vi "SQL查询.vi"(7 "condition":string, 10 "table输入":string(combo), 11 "database":string(combo)) -> (0 "error out":errorcluster, 3 "data":string[][](table))   [LabVIEW 2016, in "数据传输系统.lvlib"]
uses:
  <vilib>/Utility/sysdir.llb/System Directory Type.ctl
  <vilib>/addons/database/Connection.llb/DB Tools Open Connec (String).vi
  <vilib>/addons/database/_DB Variant To Data/Database Variant To Data.xnode
  <vilib>/addons/database/NI_Database_API.lvlib
panel:
  out "子数组":string[](array[string])
  in  "error in (no error)":errorcluster
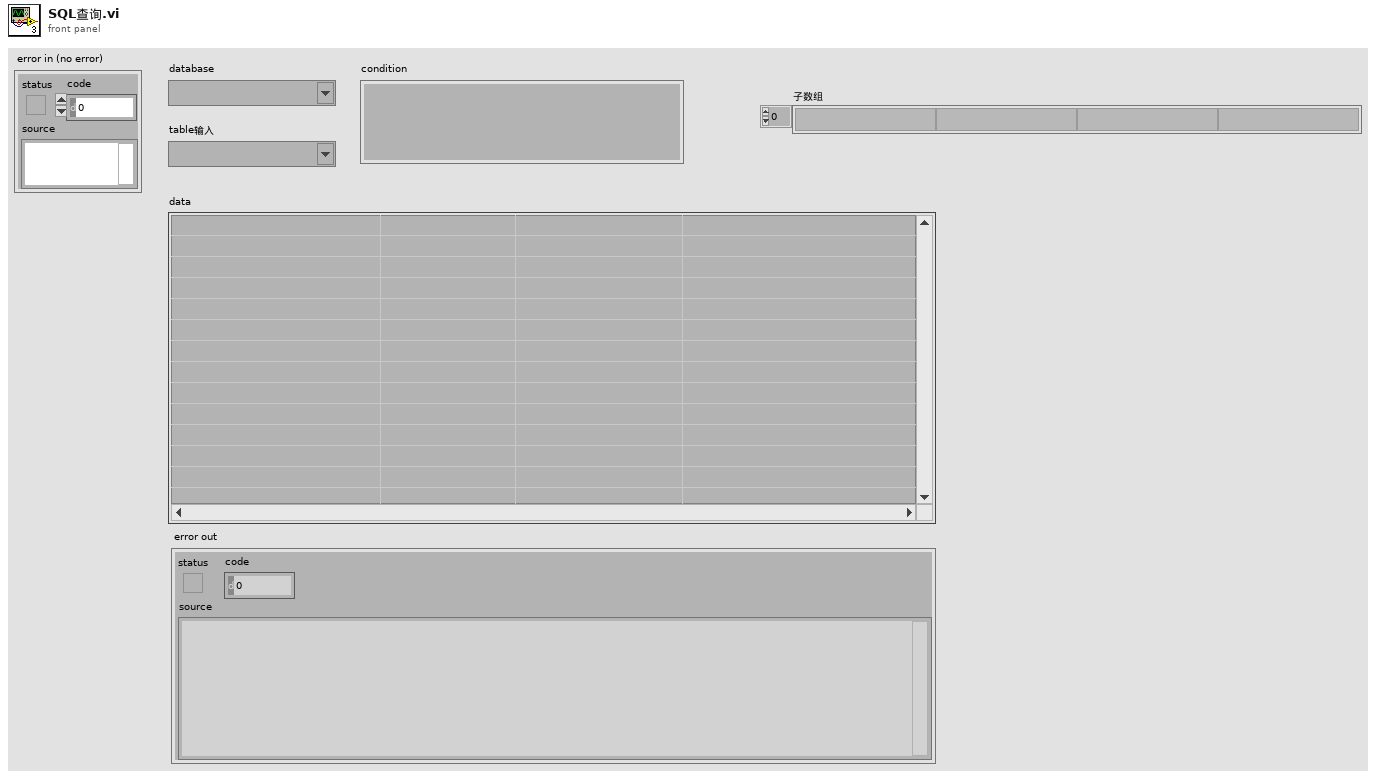
[diagram p1: front panel]
types:
  T1 = typedef "System Directory Type.ctl" = i32
  T2 = typedef "NI_Database_API.lvlib/Conn ObjectReference.ctl" = refnum<k1>
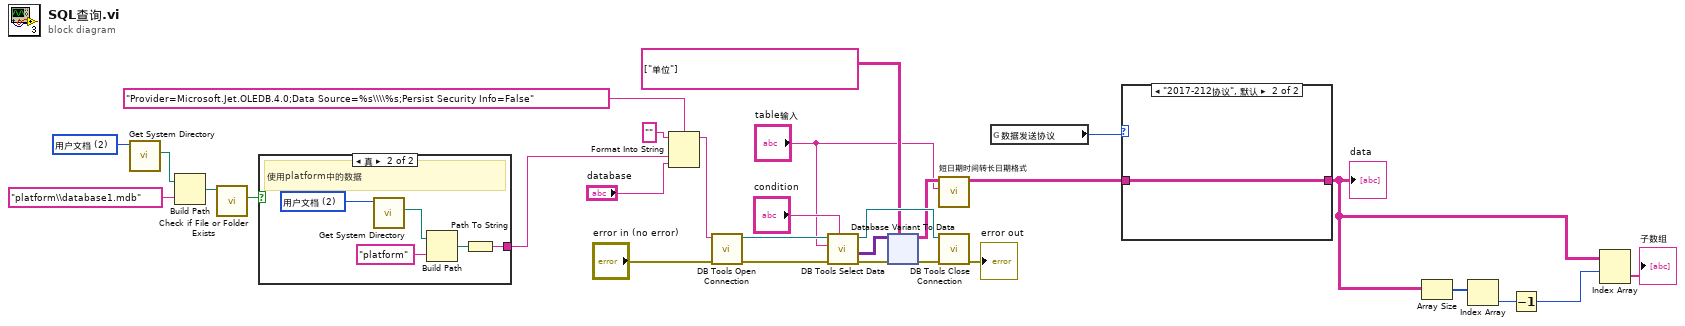
[diagram p0: block diagram]
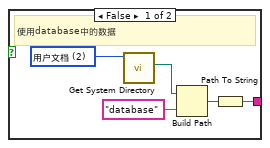
[diagram p2: hidden frame]
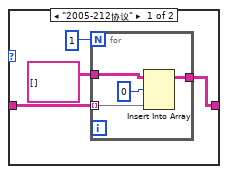
[diagram p3: hidden frame]
diagram:
  w5 = T1 2 items=["用户目录"=0, "用户桌面"=1, "用户文档"=2, "用户应用程序数据"=3, "用户设置"=4, "用户临时目录"=5, "公共文档"=6, "公共应用程序数据"=7, "公共设置"=8, "公共缓存"=13, "系统核心库"=9, "系统安装库"=10, "应用程序文件"=11, "启动盘根目录"=12] ("system directory type")
  n1 = call <vilib>:"Get System Directory.vi"("system directory type"=w5) -> ("system directory"=w6:path)  [unwired: 10 in]
  n2 = Build Path(base path=w6, name or relative path="platform\\database1.mdb" ("condition")) -> (appended path=w4:path)
  n3 = call <vilib>:"Check if File or Folder Exists.vi"("path"=w4) -> ("file or folder exists?"=w2:bool)  [unwired: 8 in, 2 out]
  n4 = case shown="真" w2 {
    tunnel: [w30 w35] -> w1
    frame False {
      w33 = T1 2 items=["用户目录"=0, "用户桌面"=1, "用户文档"=2, "用户应用程序数据"=3, "用户设置"=4, "用户临时目录"=5, "公共文档"=6, "公共应用程序数据"=7, "公共设置"=8, "公共缓存"=13, "系统核心库"=9, "系统安装库"=10, "应用程序文件"=11, "启动盘根目录"=12] ("system directory type")
      # "使用database中的数据"
      n5 = call <vilib>:"Get System Directory.vi"("system directory type"=w33) -> ("system directory"=w32:path)  [unwired: 10 in]
      n6 = Build Path(base path=w32, name or relative path="database" ("condition")) -> (appended path=w34:path)
      n7 = Path To String(path=w34) -> (string=w30:string)
    }
    frame True {
      w39 = T1 2 items=["用户目录"=0, "用户桌面"=1, "用户文档"=2, "用户应用程序数据"=3, "用户设置"=4, "用户临时目录"=5, "公共文档"=6, "公共应用程序数据"=7, "公共设置"=8, "公共缓存"=13, "系统核心库"=9, "系统安装库"=10, "应用程序文件"=11, "启动盘根目录"=12] ("system directory type")
      # "使用platform中的数据"
      n8 = call <vilib>:"Get System Directory.vi"("system directory type"=w39) -> ("system directory"=w38:path)  [unwired: 10 in]
      n9 = Build Path(base path=w38, name or relative path="platform" ("condition")) -> (appended path=w36:path)
      n10 = Path To String(path=w36) -> (string=w35:string)
    }
  }
  n11 = Format Into String(format string="Provider=Microsoft.Jet.OLEDB.4.0;Data Source=%s\\\\%s;Persist Security Info=False" ("格式字符串"), initial string="" ("初始字符串"), w1, "database") -> (resulting string=w18:string)  [unwired: 1 in, 1 out]
  n12 = call-poly <vilib>:"DB Tools Open Connection.vi"("error in (no error)"="error in (no error)", "connection information"=w18) -> ("error out"=w16:errorcluster, "connection reference"=w17:T2)  [unwired: 6 in]
  n13 = call <vilib>:"DB Tools Select Data.vi"("condition"="condition", "error in (no error)"=w16, "table"="table输入", "connection reference"=w17) -> ("error out"=w23:errorcluster, "data"=w28:variant[][], "connection reference out"=w29:T2)  [unwired: 2 in]
  n14 = xnode "Database Variant To Data"("database variant"=w28, "error in (no error)"=w23, "type"=string[][] [["单位"]]) -> ("data"=w15:string[][], "error out"=w22:errorcluster)
  n15 = call "短日期时间转长日期格式.vi"("table输入"="table输入", "data"=w15) -> ("输出数组"=w13:string[][])  [unwired: 9 in]
  n16 = call <vilib>:"DB Tools Close Connection.vi"("error in (no error)"=w22, "connection reference"=w29) -> ("error out"=→"error out":errorcluster)  [unwired: 5 in]
  n17 = global read "断电保存全局.vi" "数据发送协议"() -> (w12:enum16{"2005-212协议", "2017-212协议"})
  n18 = case shown="\"2017-212协议\", 默认" w12 {
    tunnel: w13 -> [w41 w48]
    tunnel: [w40 w48] -> w10
    frame "2005-212协议" {
      n19 = for {
        N: 1 -> [_]
        tunnel: string[][] [] ("data") -> [w47]
        tunnel: w41 -> [w46] mode=indexing
        tunnel: [w44] -> w40
        n20 = Insert Into Array(array=w47, index (row)=0 ("索引 (行)"), new element=w46) -> (w44:string[][])  [unwired: 1 in]
      }
    }
    frame "2017-212协议", Default {
    }
  }
  "data" <- w10
  n21 = Array Size(array=w10) -> (size(s)=w11:i32[])
  n22 = Index Array(array=w11) -> (element=w8:i32)  [unwired: 1 in]
  n23 = Decrement(x=w8) -> (x-1=w7:i32)
  n24 = Index Array(array=w10, index (row)=w7) -> (element=→"子数组":string[])  [unwired: 1 in]
